vi "delete empty channel.vi"(11 "通道信息":string[][](table)) -> (3 "通道信息输出":string[][](table))   [LabVIEW 2024]
panel:
  out "Boolean":bool
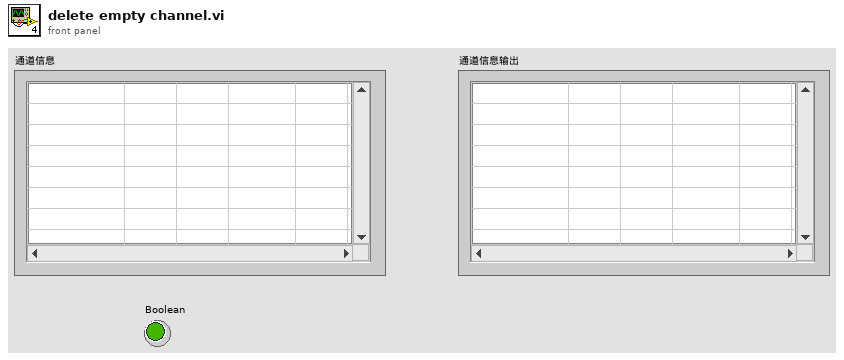
[diagram p1: front panel]
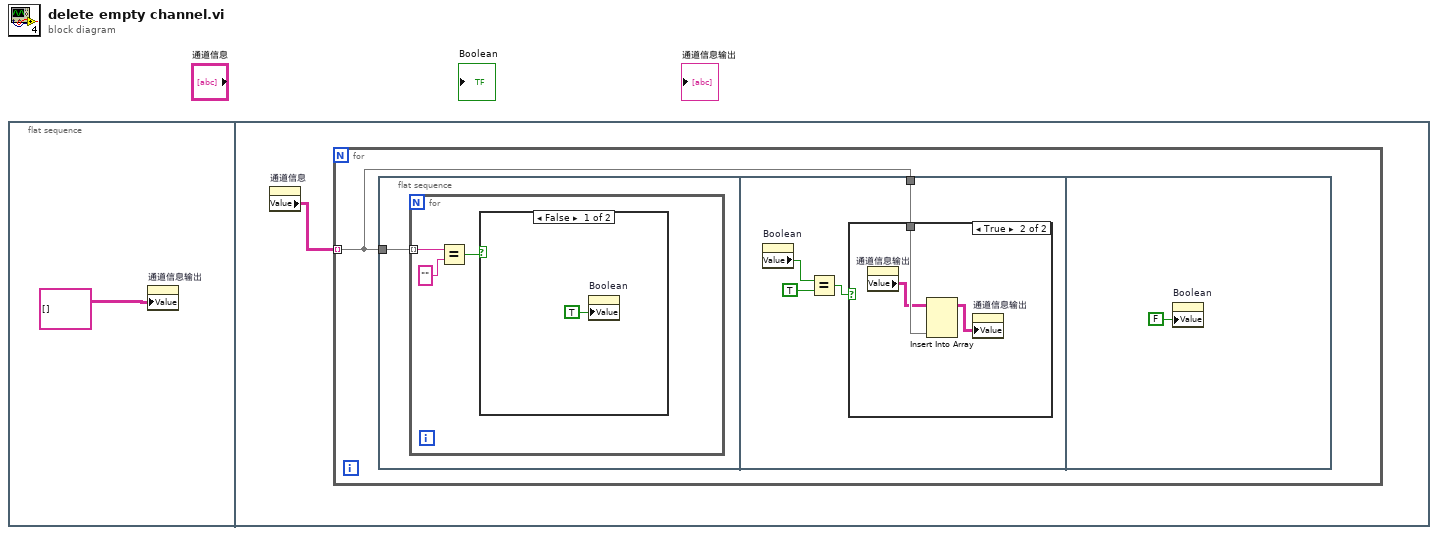
[diagram p0: block diagram]
diagram:
  n1 = flat-sequence {
    frame #0 {
      n2 = property on="通道信息输出" class="Tbl (strict)"("Value"=string[][] []) -> ()  [unwired: 2 in, 2 out]
    }
    frame #1 {
      n3 = property on="通道信息" class="Tbl (strict)"() -> ("Value"=w2:string[][])  [unwired: 2 in, 2 out]
      n4 = for {
        tunnel: w2 -> [w3] mode=indexing
        n5 = flat-sequence {
          tunnel: w3 -> [w4]
          tunnel: w3 -> [w9]
          frame #0 {
            n6 = for {
              tunnel: w4 -> [w7] mode=indexing
              n7 = Equal?(x=w7, y="") -> (x = y?=w5:bool)
              n8 = case shown="False" w5 {
                frame False {
                  n9 = property on="Boolean" class="Bool (strict)"("Value"=TRUE ("Boolean")) -> ()  [unwired: 2 in, 2 out]
                }
                frame True {
                }
              }
            }
          }
          frame #1 {
            n10 = property on="Boolean" class="Bool (strict)"() -> ("Value"=w12:bool)  [unwired: 2 in, 2 out]
            n11 = Equal?(x=w12, y=TRUE) -> (x = y?=w10:bool)
            n12 = case shown="True" w10 {
              tunnel: w9 -> [_ w15]
              frame False {
              }
              frame True {
                n13 = property on="通道信息输出" class="Tbl (strict)"() -> ("Value"=w14:string[][])  [unwired: 2 in, 2 out]
                n14 = Insert Into Array(array=w14, new element=w15) -> (w13:string[][])  [unwired: 2 in]
                n15 = property on="通道信息输出" class="Tbl (strict)"("Value"=w13) -> ()  [unwired: 2 in, 2 out]
              }
            }
          }
          frame #2 {
            n16 = property on="Boolean" class="Bool (strict)"("Value"=FALSE ("Boolean")) -> ()  [unwired: 2 in, 2 out]
          }
        }
      }
    }
  }
